vi "Matrix_ExtractMatrix.vi"(6 "StopColumnPlus1":i32, 8 "StartingColumn":i32, 9 "StopRowPlus1":i32, 10 "StartingRow":i32, 11 "input matrix":T1) -> (3 "output column":T1)   [LabVIEW 2019, in "Trajectory_Library.lvlib"]
doc: "Creates a new LINEAR SYSTEM data cluster with the specified values. \n\n\nInputs: \n - XXX -- XXX.\n\nOutputs:\n - XXX -- XXX."
uses:
  Trajectory_Library.lvlib
  <vilib>/Analysis/Matrix/Datatypes/RealMatrix.ctl
  <vilib>/Analysis/Matrix/NI_Matrix.lvlib
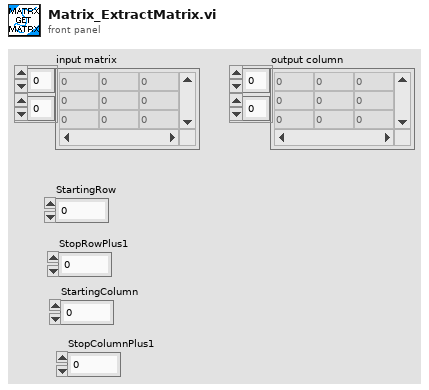
[diagram p1: front panel]
types:
  T1 = typedef "NI_Matrix.lvlib/RealMatrix.ctl" = dbl[][]
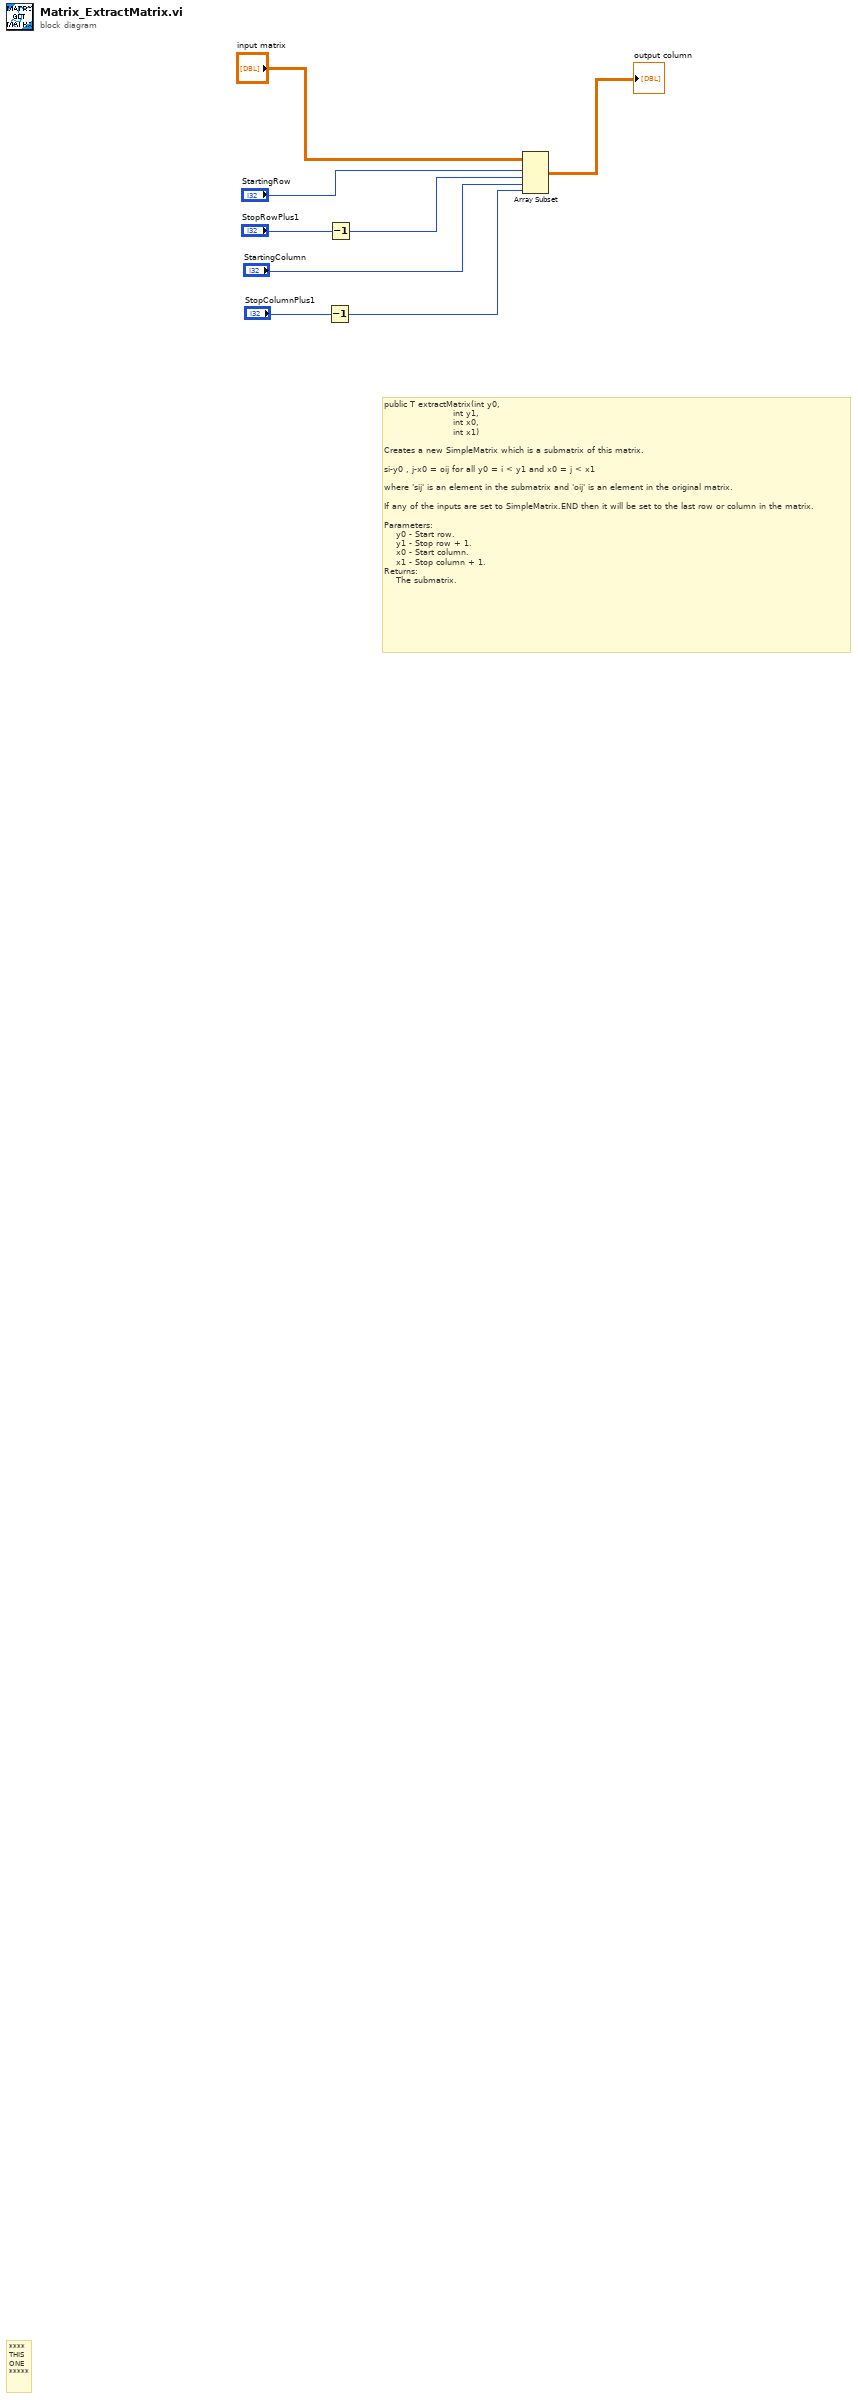
[diagram p0: block diagram]
diagram:
  # "public T extractMatrix(int y0,\n                       int y1,\n                       int x0,\n                       int x1)\n\nCreates a new SimpleMatrix which is a submatrix of this matrix.\n\nsi-y0 , j-x0 = oij for all y0 = i < y1 and x0 = j < x1\n\nwhere 'sij' is an element in the submatrix and 'oij' is an element in the original matrix.\n\nIf any of the inputs are set to SimpleMatrix.END then it will be set to the last row or column in the matrix.\n\nParameters:\n    y0 - Start row.\n    y1 - Stop row + 1.\n    x0 - Start column.\n    x1 - Stop column + 1.\nReturns:\n    The submatrix."
  # "****\nTHIS\nONE\n*****"
  n1 = Decrement(x="StopColumnPlus1") -> (x-1=w2:i32)
  n2 = Decrement(x="StopRowPlus1") -> (x-1=w1:i32)
  n3 = Array Subset(array="input matrix", index (row)="StartingRow", length (row)=w1, index (col)="StartingColumn", length (col)=w2) -> (→"output column":T1)
